vi "Generate Simulated AI Data.vi"(8 "error in":errorcluster, 10 "SimRange":cluster{"hi":dbl, "lo":dbl}, 11 "IONames[]":string[](array[string])) -> (0 "error out":errorcluster, 1 "timestamp":dbl, 2 "data":dbl[][](array[numeric]) format="%0.2f", 5 "Q element":T1)   [LabVIEW 2017, in "DAQ.lvclass"]
doc: "Developed by Kevin Thompson\nkevin@thompsonengineering.net\n\nCopyright 2018-2020\nThompson Engineering, LLC"
uses:
  DAQ.lvclass
  TD local raw AI Data--cluster.ctl
  <userlib>/_OpenG.lib/numeric/numeric.llb/Random Number Within Range - DBL__ogtk.vi
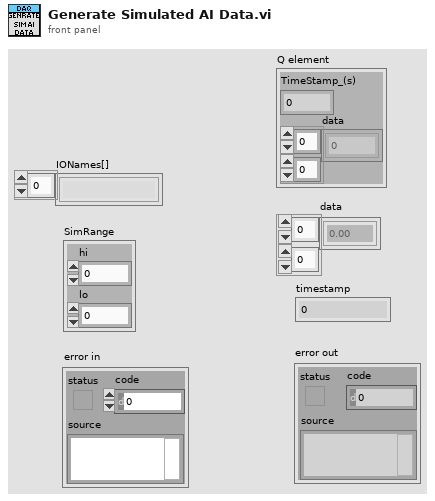
[diagram p1: front panel]
types:
  T1 = typedef "DAQ.lvclass/TD local raw AI Data--cluster.ctl" = cluster{"TimeStamp_(s)":dbl, "data":dbl[][]}
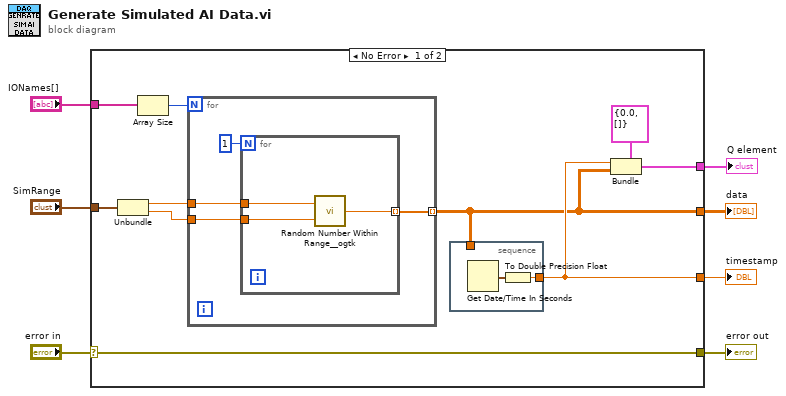
[diagram p0: block diagram]
diagram:
  n1 = case shown="No Error" "error in" {
    selector: "error in" -> [w12 w27]
    tunnel: [w9 _] -> w7
    tunnel: "SimRange" -> [w17 _]
    tunnel: [w10 _] -> w5
    tunnel: "IONames[]" -> [w13 _]
    tunnel: [w12 w27] -> w2
    tunnel: [w8 _] -> w1
    frame No Error {
      n2 = Unbundle(w17) -> ("hi"=w16:dbl, "lo"=w15:dbl)
      n3 = Array Size(array=w13) -> (size(s)=w14:i32)
      n4 = for {
        N: w14 -> [_]
        tunnel: w16 -> [w22]
        tunnel: w15 -> [w21]
        tunnel: [w20] -> w9 mode=indexing
        n5 = for {
          N: 1 -> [_]
          tunnel: w22 -> [w26]
          tunnel: w21 -> [w25]
          tunnel: [w24] -> w20 mode=indexing
          n6 = call-poly <userlib>:"Random Number Within Range__ogtk.vi"("High"=w26, "Low"=w25) -> ("Random Number"=w24:dbl)  [unwired: 3 in]
        }
      }
      n7 = stacked-sequence {
        tunnel: [w18] -> w10
        tunnel: w9 -> [_]
        frame #0 {
          n8 = Get Date/Time In Seconds() -> (seconds since 1Jan1904=w19:timestamp)
          n9 = To Double Precision Float(number=w19) -> (double precision float=w18:dbl)
        }
      }
      n10 = Bundle(cluster=T1 {"TimeStamp_(s)"=0.0, "data"=[]} ("output cluster"), "TimeStamp_(s)"=w10, "data"=w9) -> (w8:T1)
    }
    frame Error {
    }
  }
  "error out" <- w2
  "data" <- w7
  "timestamp" <- w5
  "Q element" <- w1
